vi "YCBCR.vi"(4 "data 3":u8[](array[numeric]), 5 "data":u8[](array[numeric]), 6 "Numeric":i32, 7 "data 2":u8[](array[numeric]), 8 "Numeric 2":i32, 9 "Numeric 3":i32, 10 "Numeric 4":i32, 11 "data 4":u8[](array[numeric])) -> (0 "Array":u8[](array[numeric]), 1 "Cr":dbl[](array[numeric]), 2 "Cb":dbl[](array[numeric]), 3 "Y":dbl[](array[numeric]))   [LabVIEW 2012]
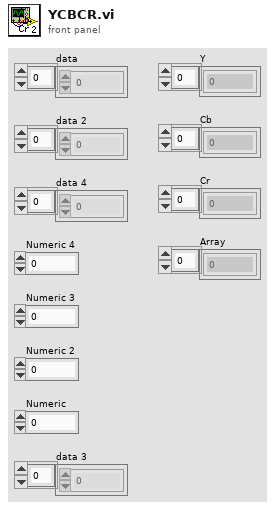
[diagram p1: front panel]
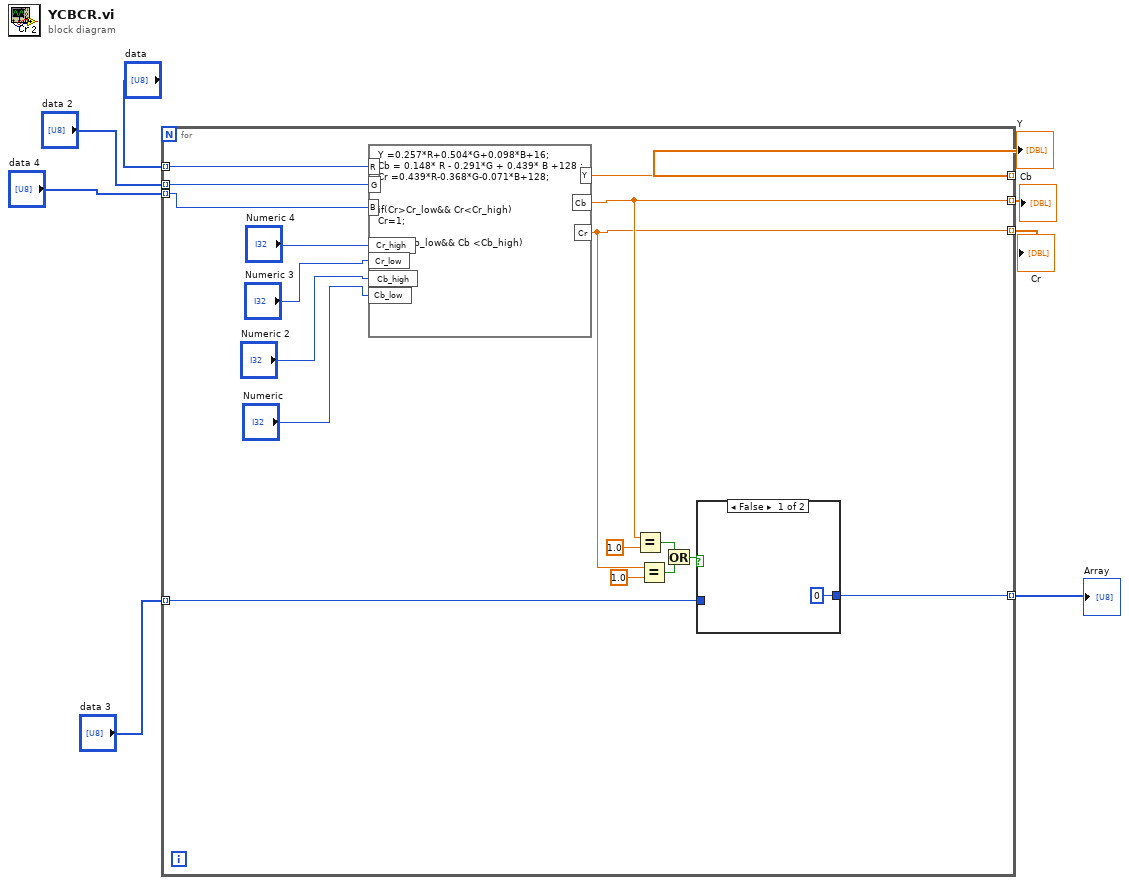
[diagram p0: block diagram]
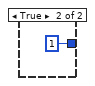
[diagram p2: hidden frame]
diagram:
  n1 = for {
    tunnel: "data 4" -> [w25] mode=indexing
    tunnel: [w22] -> w4 mode=indexing
    tunnel: [w23] -> w3 mode=indexing
    tunnel: [w24] -> w2 mode=indexing
    tunnel: "data 3" -> [w19] mode=indexing
    tunnel: [w18] -> w6 mode=indexing
    tunnel: "data 2" -> [w14] mode=indexing
    tunnel: "data" -> [w13] mode=indexing
    n2 = formula code="Y =0.257*R+0.504*G+0.098*B+16;\nCb = 0.148* R - 0.291*G + 0.439* B +128 ;\nCr =0.439*R-0.368*G-0.071*B+128;\n\n\nif(Cr>Cr_low&& Cr<Cr_high)\nCr=1;\n\nif(Cb>Cb_low&& Cb <Cb_high)\nCb =1;"("R"=w13, "G"=w14, "B"=w25, "Cr_high"="Numeric 4", "Cr_low"="Numeric 3", "Cb_high"="Numeric 2", "Cb_low"="Numeric") -> ("Y"=w24:dbl, "Cb"=w23:dbl, "Cr"=w22:dbl)
    n3 = Equal?(x=w23, y=1.0) -> (x = y?=w17:bool)
    n4 = Equal?(x=w22, y=1.0) -> (x = y?=w16:bool)
    n5 = Or(x=w17, y=w16) -> (x .or. y?=w15:bool)
    n6 = case shown="False" w15 {
      tunnel: w19 -> [_ _]
      tunnel: [u8 0 u8 1] -> w18
      frame False {
      }
      frame True {
      }
    }
  }
  "Y" <- w2
  "Cb" <- w3
  "Cr" <- w4
  "Array" <- w6
